vi "disconnect.vi"(8 "error in (no error)":errorcluster, 11 "MonoClientCommunicator in":refnum<class "MonoClientCommunicator.lvclass">) -> (0 "error out":errorcluster, 3 "MonoClientCommunicator out":refnum<class "MonoClientCommunicator.lvclass">)   [LabVIEW 2016, in "MonoClientCommunicator.lvclass"]
uses:
  MonoClientCommunicator.lvclass
  MonoClientCommunicator.lvclass/MonoClientCommunicator.ctl
  ts_labview_tcp/TCPClient/TCPClient.lvclass
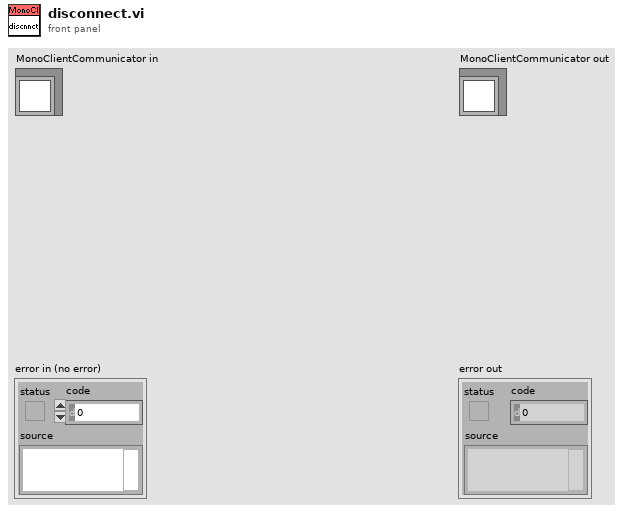
[diagram p1: front panel]
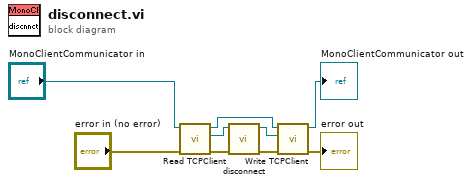
[diagram p0: block diagram]
diagram:
  n1 = call "Read TCPClient.vi"("error in (no error)"="error in (no error)", "MonoClient in"="MonoClientCommunicator in") -> ("error out"=w7:errorcluster, "TCPClient.lvclass"=w8:refnum<class "TCPClient.lvclass">, "MonoClient out"=w5:refnum<class "MonoClientCommunicator.lvclass">)  [unwired: 7 in]
  n2 = call-dynamic "disconnect.vi"("error in (no error)"=w7, "TCPClient in"=w8) -> ("error out"=w3:errorcluster, "TCPClient out"=w4:refnum<class "TCPClient.lvclass">)  [unwired: 8 in]
  n3 = call "Write TCPClient.vi"("error in (no error)"=w3, "TCPClient.lvclass"=w4, "MonoClient in"=w5) -> ("error out"=→"error out":errorcluster, "MonoClient out"=→"MonoClientCommunicator out":refnum<class "MonoClientCommunicator.lvclass">)  [unwired: 7 in]
